vi "Raster.vi"(4 "Draw Lines":bool, 6 "Line Colour":u32(colorbox)=4375295, 10 "Triangles Sorted":T1[](array[typedef]), 11 "Pixels":refnum<data-value>) -> (3 "Pixels (dup)":refnum<data-value>)   [LabVIEW 2020, in "3D.lvlib"]
uses:
  3D.lvlib
  Triangle 2D.ctl
  Point 2D.ctl
  <vilib>/Utility/High Resolution Relative Seconds.vi
  Raster/Draw Flat Bottom Filled Triangle.vi
  Raster/Draw Flat Top Filled Triangle.vi
  Raster/Sort Points.vi
  Raster/Draw Horizontal Line.vi
  <userlib>/_OpenG.lib/array/array.llb/Sort Array__ogtk.vi
  <userlib>/_OpenG.lib/array/array.llb/Sort 1D Array (I32)__ogtk.vi
  Raster/Raster.lvlib
  Utility/Utility.lvlib
panel:
  out "Delta Time [s]":dbl format="%.3p"
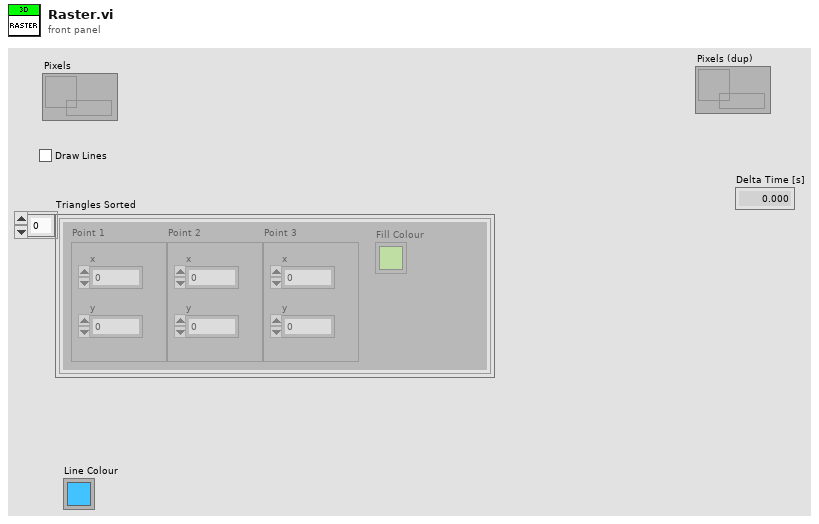
[diagram p1: front panel]
types:
  T1 = typedef "3D.lvlib/Triangle 2D.ctl" = cluster{"Point 1":T2, "Point 2":T2, "Point 3":T2, "Fill Colour":u32}
  T2 = typedef "3D.lvlib/Point 2D.ctl" = cluster{"x":sgl, "y":sgl}
  T3 = typedef "Raster.lvlib/Point 2D.ctl" = cluster{"x":i32, "y":i32}
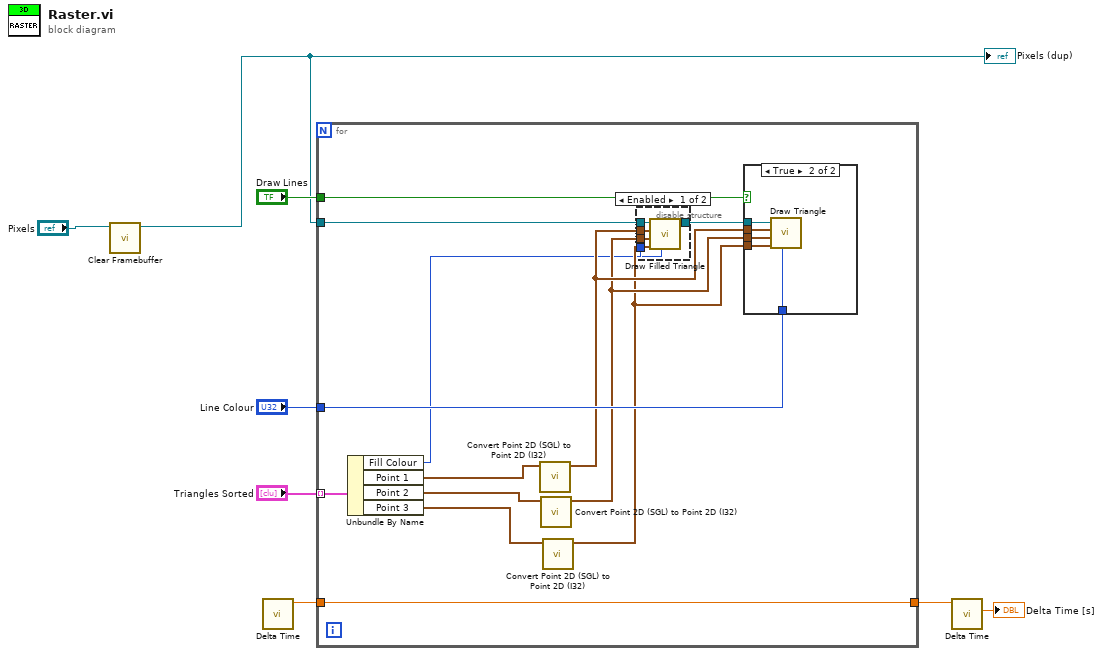
[diagram p0: block diagram]
diagram:
  n1 = call "Clear Framebuffer.vi"("Frame Buffer in"="Pixels") -> ("Frame Buffer out"=w1:refnum<data-value>)  [unwired: 10 in]
  "Pixels (dup)" <- w1
  n2 = call "Delta Time.vi"() -> ("Relative Seconds Out"=w5:dbl)  [unwired: 10 in, 1 out]
  n3 = for {
    tunnel: "Line Colour" -> [w21]
    tunnel: "Triangles Sorted" -> [w20] mode=indexing
    tunnel: "Draw Lines" -> [w12]
    tunnel: w5 -> [w11]
    tunnel: [w11] -> w4
    tunnel: w1 -> [w10]
    n4 = Unbundle By Name(w20) -> ("Fill Colour"=w13:u32, "Point 1"=w19:T2, "Point 2"=w18:T2, "Point 3"=w17:T2)
    n5 = call "Convert Point 2D (SGL) to Point 2D (I32).vi"("Point 2D (Float)"=w19) -> ("Point 2D (I32)"=w16:T3)  [unwired: 10 in]
    n6 = call "Convert Point 2D (SGL) to Point 2D (I32).vi"("Point 2D (Float)"=w18) -> ("Point 2D (I32)"=w15:T3)  [unwired: 10 in]
    n7 = call "Convert Point 2D (SGL) to Point 2D (I32).vi"("Point 2D (Float)"=w17) -> ("Point 2D (I32)"=w14:T3)  [unwired: 10 in]
    n8 = disable-structure shown="Enabled" {
      disable-tunnel: w16 -> [w27 _]
      disable-tunnel: w15 -> [w26 _]
      disable-tunnel: w14 -> [w25 _]
      disable-tunnel: w13 -> [w24 _]
      disable-tunnel: w10 -> [w23 w28]
      disable-tunnel: [w22 w28] -> w9
      frame Enabled {
        n9 = call "Draw Filled Triangle.vi"("Fill Colour"=w24, "Point 3"=w25, "Point 2"=w26, "Point 1"=w27, "Pixels in"=w23) -> ("Pixels (dup)"=w22:refnum<data-value>)  [unwired: 6 in]
      }
      frame Disabled {
      }
    }
    n10 = case shown="True" w12 {
      tunnel: w9 -> [_ w29]
      tunnel: w21 -> [_ w33]
      tunnel: w16 -> [_ w32]
      tunnel: w15 -> [_ w31]
      tunnel: w14 -> [_ w30]
      frame False {
      }
      frame True {
        n11 = call "Draw Triangle.vi"("Line Colour"=w33, "Point 3"=w30, "Point 2"=w31, "Point 1"=w32, "Pixels"=w29) -> ()  [unwired: 6 in, 1 out]
      }
    }
  }
  n12 = call "Delta Time.vi"("Relative Seconds In"=w4) -> ("Delta Time [s]"=→"Delta Time [s]":dbl)  [unwired: 9 in, 1 out]
